vi "5492_AutoLiftNoPID.vi"   [LabVIEW 2017]
uses:
  5492_LiftButtons.vi
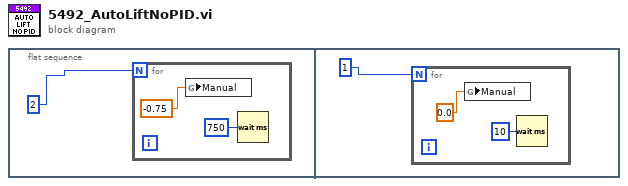
[diagram p0: block diagram]
diagram:
  n1 = flat-sequence {
    frame #0 {
      n2 = for {
        N: 2 -> [_]
        n3 = global write "5492_LiftButtons.vi" "Manual"(-0.75 ("Manual")) -> ()
        n4 = Wait (ms)(milliseconds to wait=u32 750) -> ()  [unwired: 1 out]
      }
    }
    frame #1 {
      n5 = for {
        N: 1 -> [_]
        n6 = global write "5492_LiftButtons.vi" "Manual"(0.0 ("Manual")) -> ()
        n7 = Wait (ms)(milliseconds to wait=u32 10) -> ()  [unwired: 1 out]
      }
    }
  }
